vi "Handle Error.vi"(8 "error in (no error)":errorcluster, 11 "Measure Object in":refnum<class "Template Module.lvclass">) -> (0 "error out":errorcluster, 2 "stop actor?":bool=TRUE, 3 "Measure Object out":refnum<class "Template Module.lvclass">)   [LabVIEW 2018, in "Template Module.lvclass"]
doc: "(<B>Filename</B>: Actor Framework.lvlib:Actor.lvclass:Handle Error.vi)\n\nDefines how the actor handles an error that occurred while processing a message. By default, this method does nothing except stop the actor."
uses:
  Template Module.lvclass
  C:/Program Files/National Instruments/LabVIEW 2018/vi.lib/ActorFramework/Actor/Actor.lvclass
  <vilib>/ActorFramework/Actor/Actor.lvclass/Actor.ctl
  Controllers/Application Controller Messages/Display Error Msg/Display Error Msg.lvclass/Display Error Msg.ctl
  <vilib>/ActorFramework/Message Enqueuer/Message Enqueuer.lvclass/Message Enqueuer.ctl
  <vilib>/ActorFramework/Message Enqueuer/Enqueue.vi
  <vilib>/ActorFramework/Message Enqueuer/Init from Existing Queue.vi
  Controllers/Application Controller Messages/Display Error Msg/Display Error Msg.lvclass
  C:/Program Files/National Instruments/LabVIEW 2018/vi.lib/ActorFramework/Message/Message.lvclass
  <vilib>/ActorFramework/Stop Msg/Stop Msg.lvclass
  <vilib>/ActorFramework/Message Priority Queue/Priority Enqueue.vi
  <vilib>/ActorFramework/Actor/Actor.lvclass
  <vilib>/ActorFramework/Message Enqueuer/Message Enqueuer.lvclass
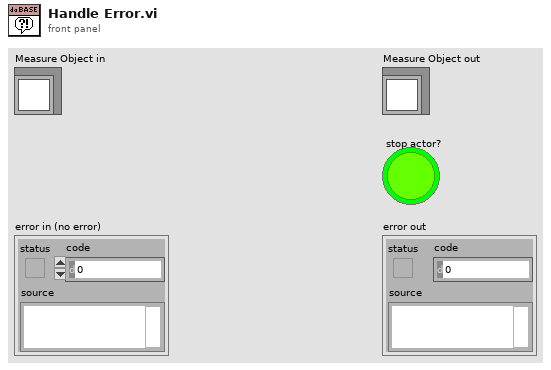
[diagram p1: front panel]
types:
  T1 = typedef "LabActor Error.ctl" = cluster{"Time":string, "Message":string, "Source":string, "Code":i32, "Error?":bool, "Module":string}
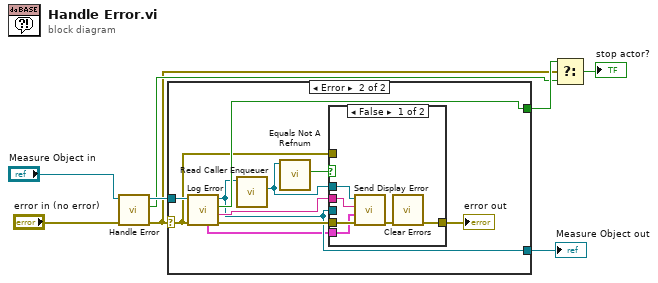
[diagram p0: block diagram]
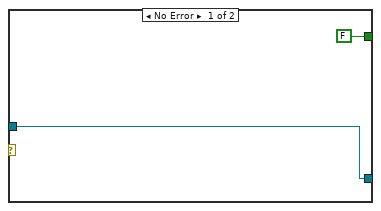
[diagram p2: hidden frame]
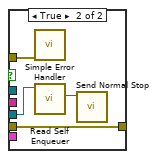
[diagram p3: hidden frame]
diagram:
  n1 = call-parent "Handle Error.vi"("error in (no error)"="error in (no error)", "Actor in"="Measure Object in") -> ("error out"=w1:errorcluster, "stop actor?"=w4:bool, "Actor out"=w6:refnum<class "Template Module.lvclass">)  [unwired: 7 in]
  n2 = case shown="Error" w1 {
    selector: w1 -> [_ w12]
    tunnel: w6 -> [w9 w20]
    tunnel: [FALSE w19] -> w5
    tunnel: [w9 w13] -> w2
    frame No Error {
    }
    frame Error {
      n3 = call-dynamic "Log Error.vi"("error in (no error)"=w12, "Da Base in"=w20) -> ("error out"=w18:errorcluster, "Error message"=w16:string, "stop actor?"=w19:bool, "Da Base out"=w13:refnum<class "Template Module.lvclass">, "LabActor Error"=w11:T1)  [unwired: 5 in]
      n4 = call <vilib>:"Read Caller Enqueuer.vi"("Actor"=w13) -> ("Caller Enqueuer"=w15:refnum<class "Message Enqueuer.lvclass">)  [unwired: 10 in]
      n5 = call <vilib>:"Equals Not A Refnum.vi"("Message Enqueuer"=w15) -> ("Not a refnum?"=w14:bool)  [unwired: 10 in]
      n6 = case shown="False" w14 {
        tunnel: w18 -> [w26 w27]
        tunnel: [w22 w27] -> w17
        tunnel: w16 -> [w24 _]
        tunnel: w15 -> [w23 _]
        tunnel: w13 -> [_ w29]
        tunnel: w12 -> [_ w28]
        tunnel: w11 -> [w21 _]
        frame False {
          n7 = call "Send Display Error.vi"("error in (no error)"=w26, "LabActor Error"=w21, "Error message"=w24, "Message Enqueuer"=w23) -> ("error out"=w25:errorcluster)  [unwired: 6 in, 1 out]
          n8 = call <vilib>:"Clear Errors.vi"("error in (no error)"=w25) -> ("error out"=w22:errorcluster)  [unwired: 5 in, 1 out]
        }
        frame True {
          n9 = call <vilib>:"Simple Error Handler.vi"("error in (no error)"=w28) -> ()  [unwired: 4 in, 5 out]
          n10 = call <vilib>:"Read Self Enqueuer.vi"("Actor"=w29) -> ("Self Enqueuer"=w30:refnum<class "Message Enqueuer.lvclass">)  [unwired: 10 in]
          n11 = call <vilib>:"Send Normal Stop.vi"("Message Enqueuer"=w30) -> ()  [unwired: 10 in, 1 out]
        }
      }
      "error out" <- w17
    }
  }
  "Measure Object out" <- w2
  n12 = Select(t=w5, s=w1, f=w4) -> (s? t:f=→"stop actor?":bool)
